vi "+S2C_Access.vi"() -> ()   [LabVIEW 2015]
uses:
  S2C_Access_Select.ctl
  S2C_Access_Globals.vi
panel:
  in  "DSN_Path":path=path "C:/Personal/Labview/S2C/AccessDB.dsn" caption="DSN File Path"
  out "Info":string caption="Database Information"
  out "TblName":string
  in  "TblSelect":T1="<Select>" caption="Table"
  in  "Table":i32(listbox) caption="Parameter Table"
  out "Err":bool
  in  "Section":T1="<Select>"
  out "Init":bool
  out "Error Out":errorcluster
  in  "Error In":errorcluster
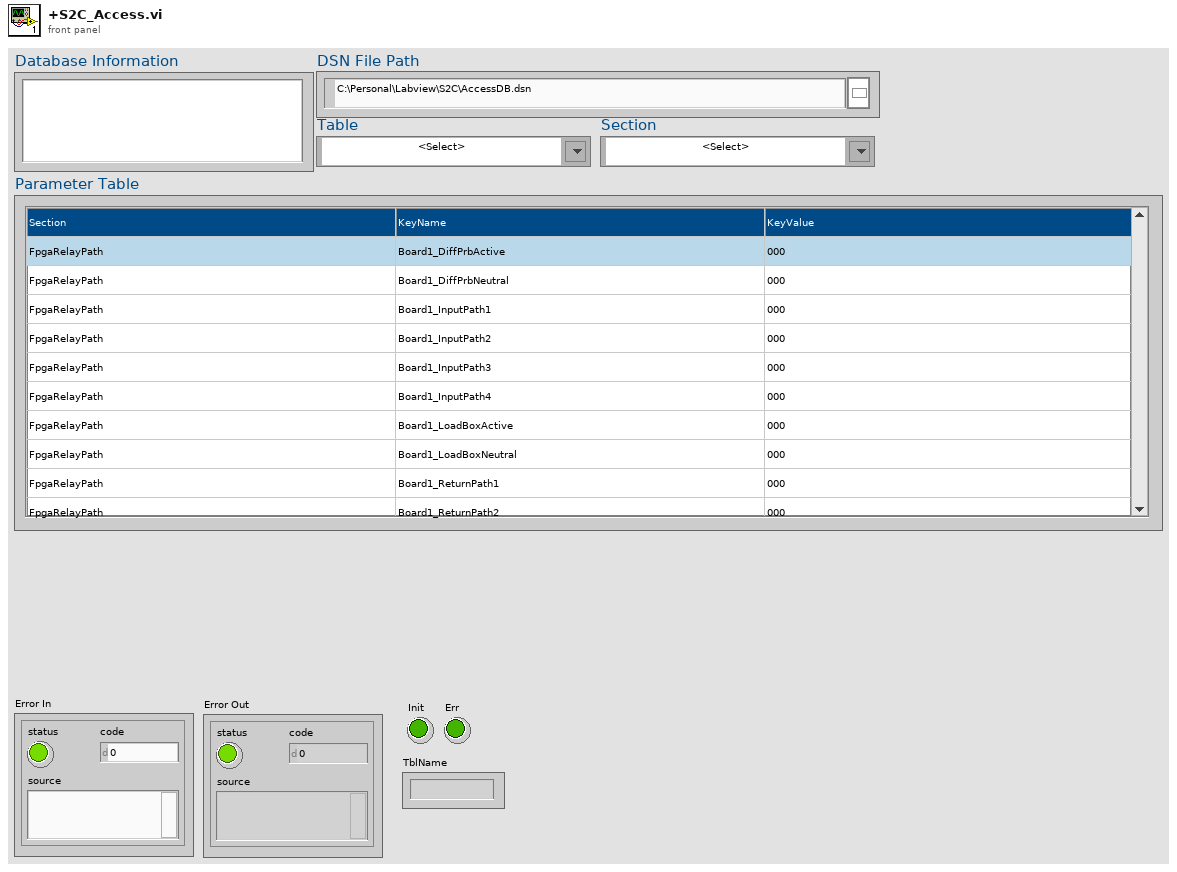
[diagram p1: front panel]
types:
  T1 = typedef "S2C_Access_Select.ctl" = string
  T2 = typedef "LVPoint32TypeDef.ctl" = cluster{"Horizontal":i32, "Vertical":i32}
  T3 = typedef "LVRowAndColumnTypeDef.ctl" = cluster{"Row":i32, "Column":i32}
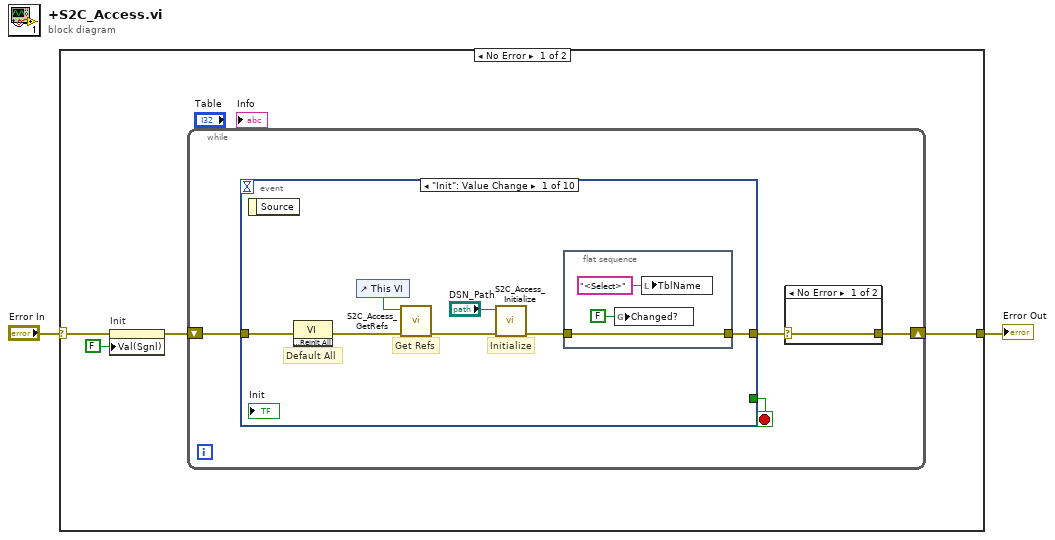
[diagram p0: block diagram]
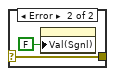
[diagram p2: hidden frame]
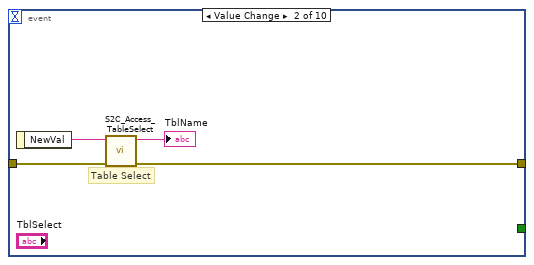
[diagram p3: hidden frame]
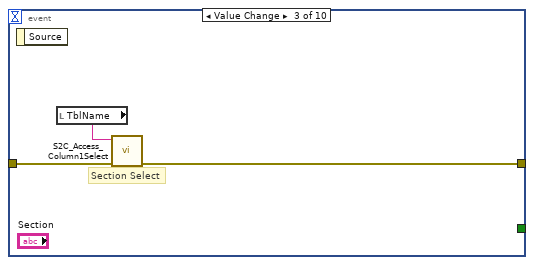
[diagram p4: hidden frame]
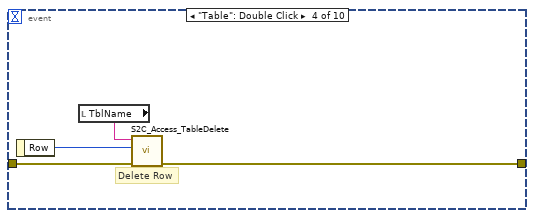
[diagram p5: hidden frame]
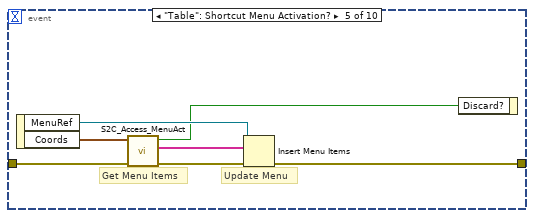
[diagram p6: hidden frame]
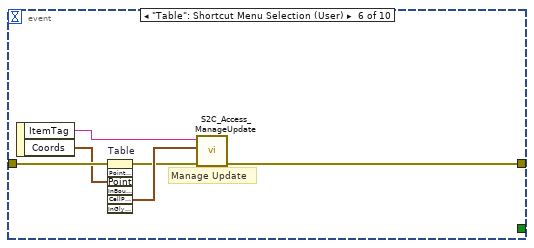
[diagram p7: hidden frame]
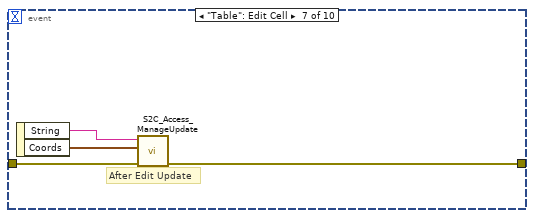
[diagram p8: hidden frame]
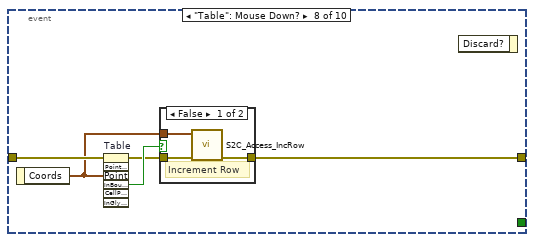
[diagram p9: hidden frame]
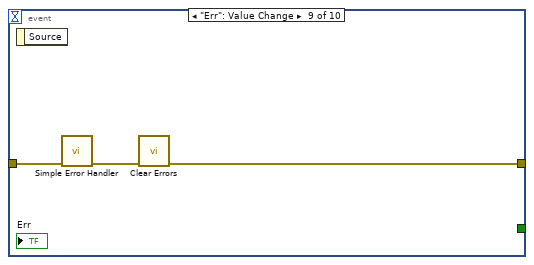
[diagram p11: hidden frame]
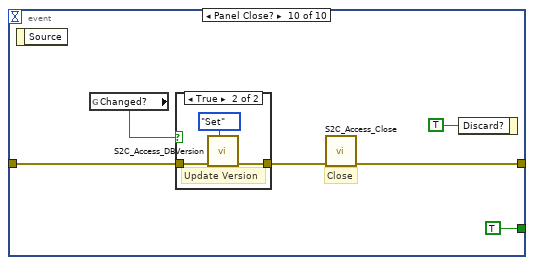
[diagram p12: hidden frame]
diagram:
  n1 = case shown="No Error" "Error In" {
    selector: "Error In" -> [w5 w74]
    tunnel: [w6 w74] -> w1
    frame No Error {
      n2 = property on="Init" class="Bool (strict)"(error in=w5, "Val(Sgnl)"=FALSE ("Value (Signaling)")) -> (error out=w4:errorcluster)  [unwired: 1 in, 1 out]
      n3 = while {
        shift-right: [w7] -> w6
        shift-left: w4 -> [w10]
        stop <- w9 stop-if-true
        n4 = event shown="[0] \"Init\": Value Change" {
          selector: _ -> [_ _ _ _ _ _ _ _ _ _]
          dyn-events: _ -> [_ _ _ _ _ _ _ _ _ _]
          timeout: _ -> [_ _ _ _ _ _ _ _ _ _]
          tunnel: w10 -> [w20 w27 w29 w34 w41 w47 w50 w55 w63 w66]
          tunnel: [w15 w25 w30 w33 w35 w44 w51 w56 w61 w68] -> w8
          tunnel: [_ _ _ _ _ _ _ _ _ TRUE] -> w9
          event "Init": Value Change {
            # "Initialize"
            # "Get Refs"
            # "Default All"
            n5 = event-data() -> ()  [unwired: 1 in, 1 out]
            n6 = invoke class="VI" method="Default Vals.Reinit All"(error in=w20) -> (error out=w19:errorcluster)  [unwired: 2 in, 2 out]
            n7 = control-ref of="This VI"() -> (w17:refnum<vi>)
            n8 = call "S2C_Access_GetRefs.vi"("Error In"=w19, "VI Ref"=w17) -> ("Error Out"=w18:errorcluster)  [unwired: 9 in]
            n9 = call "S2C_Access_Initialize.vi"("Error In"=w18, "DSN Path"="DSN_Path") -> ("Error Out"=w16:errorcluster)  [unwired: 9 in]
            n10 = flat-sequence {
              tunnel: w16 -> [w23]
              tunnel: [w23] -> w15
              frame #0 {
                n11 = global write "S2C_Access_Globals.vi" "Changed?"(FALSE ("Changed?")) -> ()
                n12 = local write "TblName"("<Select>" ("TblName")) -> ()
              }
            }
          }
          event Value Change {
            # "Table Select"
            n13 = event-data() -> ("NewVal"=w26:T1)  [unwired: 1 in]
            n14 = call "S2C_Access_TableSelect.vi"("Error In"=w27, "Table In"=w26) -> ("Error Out"=w25:errorcluster, "Table Out"=→"TblName":string)  [unwired: 8 in]
          }
          event Value Change {
            # "Section Select"
            n15 = event-data() -> ()  [unwired: 1 in, 1 out]
            n16 = local read "TblName"() -> (w28:string)
            n17 = call "S2C_Access_Column1Select.vi"("Error In"=w29, "Table"=w28) -> ("Error Out"=w30:errorcluster)  [unwired: 9 in]
          }
          event "Table": Double Click {
            # "Delete Row"
            n18 = event-data() -> ("Row"=w32:i32)  [unwired: 1 in]
            n19 = local read "TblName"() -> (w31:string)
            n20 = call "S2C_Access_TableDelete.vi"("Error In"=w34, "Row"=w32, "Table"=w31) -> ("Error Out"=w33:errorcluster)  [unwired: 8 in]
          }
          event "Table": Shortcut Menu Activation? {
            # "Update Menu"
            # "Get Menu Items"
            n21 = event-data() -> ("MenuRef"=w38:refnum<k9>, "Coords"=w40:T2)  [unwired: 1 in]
            n22 = call "S2C_Access_MenuAct.vi"("Error In"=w41, "Coords"=w40) -> ("Error Out"=w39:errorcluster, "MenuItems"=w37:string[], "Discard?"=w36:bool)  [unwired: 7 in]
            n23 = Insert Menu Items(6:w39, 8:w37, 9:w38) -> (0:w35:errorcluster)  [unwired: 3 in, 2 out]
            n24 = event-data("Discard?"=w36) -> ()  [unwired: 1 in, 1 out]
          }
          event "Table": Shortcut Menu Selection (User) {
            # "Manage Update"
            n25 = event-data() -> ("ItemTag"=w45:string, "Coords"=w46:T2)  [unwired: 1 in]
            n26 = invoke on="Table" class="MCListbox (strict)" method="Point To Row Column"(error in=w47, "Point"=w46) -> (error out=w42:errorcluster, "CellPosition"=w43:T3)  [unwired: 5 in, 5 out]
            n27 = call "S2C_Access_ManageUpdate.vi"("Error In"=w42, "Coords"=w43, "ItemTag"=w45) -> ("Error Out"=w44:errorcluster)  [unwired: 8 in]
          }
          event "Table": Edit Cell {
            # "After Edit Update"
            n28 = event-data() -> ("String"=w48:string, "Coords"=w49:T3)  [unwired: 1 in]
            n29 = call "S2C_Access_ManageUpdate.vi"("Error In"=w50, "Coords"=w49, "ItemTag"=w48) -> ("Error Out"=w51:errorcluster)  [unwired: 8 in]
          }
          event "Table": Mouse Down? {
            n30 = event-data() -> ("Coords"=w52:T2)  [unwired: 1 in]
            n31 = invoke on="Table" class="MCListbox (strict)" method="Point To Row Column"(error in=w55, "Point"=w52) -> (error out=w53:errorcluster, "InBounds"=w54:bool)  [unwired: 5 in, 5 out]
            n32 = case shown="False" w54 {
              tunnel: [w59 w60] -> w56
              tunnel: w53 -> [w58 w60]
              tunnel: w52 -> [w57 _]
              frame False {
                # "Increment Row"
                n33 = call "S2C_Access_IncRow.vi"("Error In"=w58, "Coords"=w57) -> ("Error Out"=w59:errorcluster)  [unwired: 9 in]
              }
              frame True {
              }
            }
            n34 = event-data() -> ()  [unwired: 2 in, 1 out]
          }
          event "Err": Value Change {
            n35 = event-data() -> ()  [unwired: 1 in, 1 out]
            n36 = call <vilib>:"Simple Error Handler.vi"("error in (no error)"=w63) -> ("error out"=w62:errorcluster)  [unwired: 4 in, 4 out]
            n37 = call <vilib>:"Clear Errors.vi"("error in (no error)"=w62) -> ("error out"=w61:errorcluster)  [unwired: 5 in, 1 out]
          }
          event Panel Close? {
            # "Close"
            n38 = event-data() -> ()  [unwired: 1 in, 1 out]
            n39 = global read "S2C_Access_Globals.vi" "Changed?"() -> (w64:bool)
            n40 = case shown="True" w64 {
              tunnel: w66 -> [w70 w73]
              tunnel: [w70 w72] -> w65
              frame False {
              }
              frame True {
                # "Update Version"
                n41 = call "S2C_Access_DBVersion.vi"("Action"=enum16{"Get", "Set"}."Set", "Error In"=w73) -> ("Error Out"=w72:errorcluster)  [unwired: 8 in, 1 out]
              }
            }
            n42 = call "S2C_Access_Close.vi"("Error In"=w65) -> ("Error Out"=w68:errorcluster)  [unwired: 10 in]
            n43 = event-data("Discard?"=TRUE) -> ()  [unwired: 1 in, 1 out]
          }
        }
        n44 = case shown="No Error" w8 {
          selector: w8 -> [w11 w13]
          tunnel: [w11 w13] -> w7
          frame No Error {
          }
          frame Error {
            n45 = property on="Err" class="Bool (strict)"("Val(Sgnl)"=FALSE ("Value (Signaling)")) -> ()  [unwired: 2 in, 2 out]
          }
        }
      }
    }
    frame Error {
    }
  }
  "Error Out" <- w1
